vi "Trim Array.vi"(11 "closeList":i32[](array[numeric])) -> (3 "Array":i32[](array[numeric]))   [LabVIEW 2015, in "Route Manager.lvclass"]
uses:
  Route Manager.lvclass
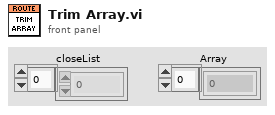
[diagram p1: front panel]
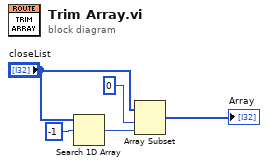
[diagram p0: block diagram]
diagram:
  n1 = Search 1D Array(1D array="closeList", element=-1) -> (index of element=w3:i32)  [unwired: 1 in]
  n2 = Array Subset(array="closeList", index=0, length=w3) -> (→"Array":i32[])
